vi "trajectory_generator.vi"(0 "T":dbl) -> (1 "Ed":dbl[](array[numeric]), 2 "Wd":dbl[](array[numeric]), 3 "Wd_dot":dbl[](array[numeric]))   [LabVIEW 2018]
uses:
  <vilib>/imath/engines/lvmath2/RunTimeEngine/IndexRead/NIMS V(S).vi
  <instcachedir>/0/NIMS V(S)_0488751826AF41519A22953C041130DC.lvgen/NIMS V(S)_0488751826AF41519A22953C041130DC_000.vi
  <vilib>/imath/engines/lvmath2/RunTimeEngine/ErrorHandling/NIMS_Create Error From Enums.vi
  <vilib>/imath/engines/lvmath2/RunTimeEngine/ArithmeticOperatorToken/NIMS_ArithmeticOperator_multmx(M,CV)-internal.vi
  <instcachedir>/0/NIMS_ArithmeticOperator_multmx(M,CV)-internal_5287250D8D1D4A3E9F77F5DF08D432E0.lvgen/NIMS_ArithmeticOperator_multmx(M,CV)-internal_5287250D8D1D4A3E9F77F5DF08D432E0_001.vi
  <vilib>/imathl/engines/lvmath/Functions/Error Handling/Create Error.vi
  <vilib>/imath/engines/lvmath2/RunTimeEngine/NodeEndStatement/NIMS_NodeEndStatement_Output.vi
  <instcachedir>/0/NIMS_NodeEndStatement_Output_53EC0D466D134D7ABD903AC30B43404B.lvgen/NIMS_NodeEndStatement_Output_53EC0D466D134D7ABD903AC30B43404B_005.vi
  <vilib>/imath/engines/lvmath2/RunTimeEngine/ErrorHandling/NIMS_Finalize Error.vi
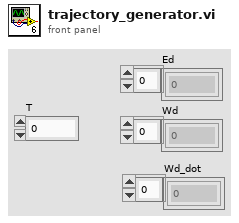
[diagram p1: front panel]
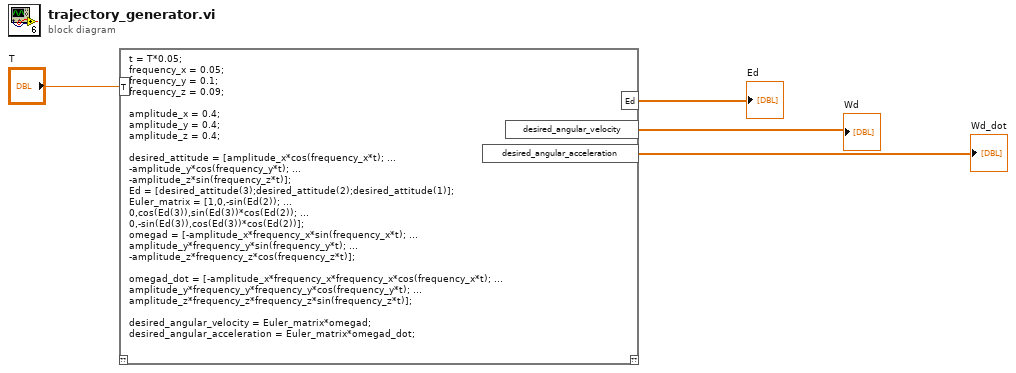
[diagram p0: block diagram]
diagram:
  n1 = mathscript code="t = T*0.05;\nfrequency_x = 0.05;\nfrequency_y = 0.1;\nfrequency_z = 0.09;\n\namplitude_x = 0.4;\namplitude_y = 0.4;\namplitude_z = 0.4;\n\ndesired_attitude = [amplitude_x*cos(frequency_x*t); ...\n-amplitude_y*cos(frequency_y*t); ...\n-amplitude_z*sin(frequency_z*t)];\nEd = [desired_attitude(3);desired_attitude(2);desired_attitude(1)];\nEuler_matrix = [1,0,-sin(Ed(2)); ...\n0,cos(Ed(3)),sin(Ed(3))*cos(Ed(2)); ...\n0,-sin(Ed(3)),cos(Ed(3))*cos(Ed(2))];\nomegad = [-amplitude_x*frequency_x*sin(frequency_x*t); ...\namplitude_y*frequency_y*sin(frequency_y*t); ...\n-amplitude_z*frequency_z*cos(frequency_z*t)];\n\nomegad_dot = [-amplitude_x*frequency_x*frequency_x*cos(frequency_x*t); ...\namplitude_y*frequency_y*frequency_y*cos(frequency_y*t); ...\namplitude_z*frequency_z*frequency_z*sin(frequency_z*t)];\n\ndesired_angular_velocity = Euler_matrix*omegad;\ndesired_angular_acceleration = Euler_matrix*omegad_dot;"("T"="T") -> ("desired_angular_velocity"=→"Wd":dbl[], "desired_angular_acceleration"=→"Wd_dot":dbl[], "Ed"=→"Ed":dbl[])  [unwired: 1 in, 1 out]
